vi "Get_Length_of_Tracks-2.vi"(0 "[IN] Grouped Tracks":dbl[][](array[numeric])) -> (1 "[OUT] Tracks Length\nin the Group":u16[](array[numeric]), 2 "[OUT] Single duration \ntrack exists in this\ngroup of tracks":bool, 3 "[OUT] Indexes of single \nframe tracks in the group":i32[](array[numeric]))   [LabVIEW 2013]
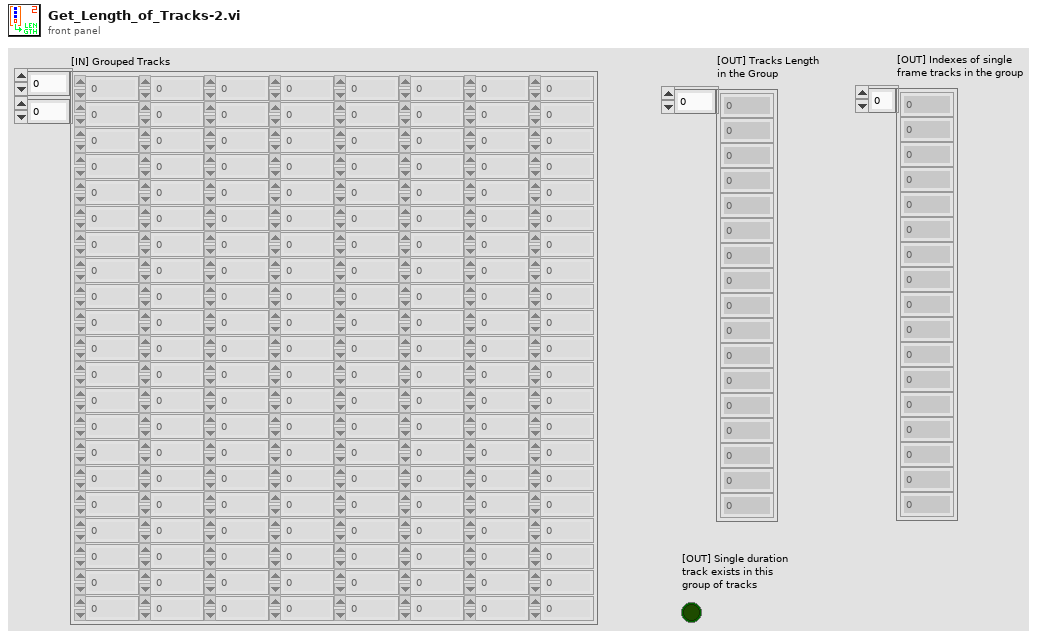
[diagram p1: front panel]
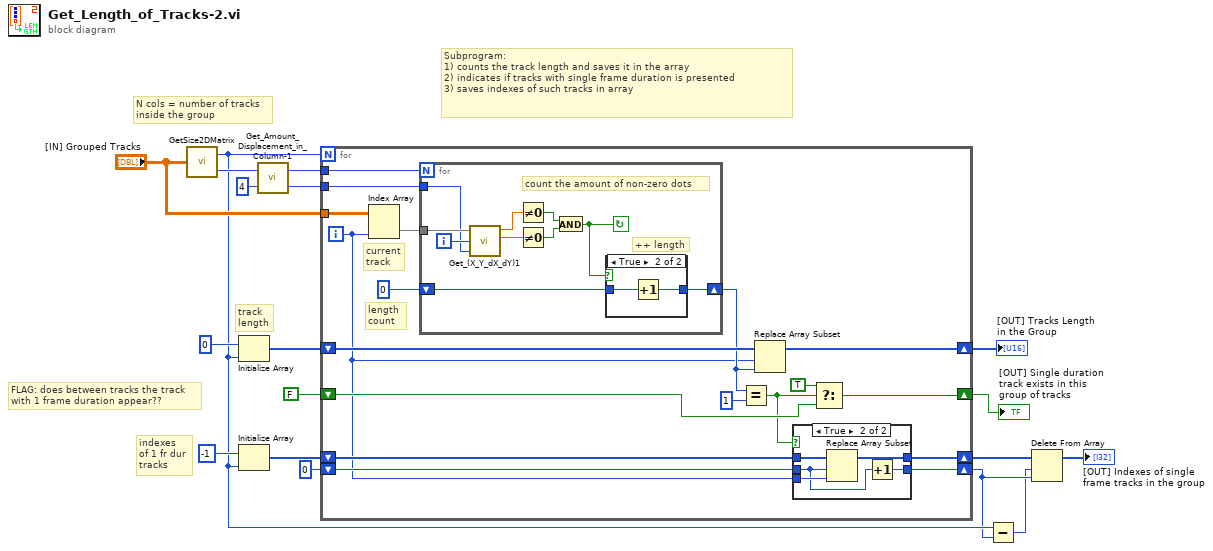
[diagram p0: block diagram]
diagram:
  # "Subprogram: \n1) counts the track length and saves it in the array\n2) indicates if tracks with single frame duration is presented\n3) saves indexes of such tracks in array"
  # "indexes \nof 1 fr dur\ntracks"
  # "FLAG: does between tracks the track \nwith 1 frame duration appear??"
  # "track \nlength"
  # "N cols = number of tracks \ninside the group"
  n1 = call "GetSize2DMatrix.vi"("Array IN (2D)"="[IN] Grouped Tracks") -> ("# Cols"=w4:i32, "# Rows"=w16:i32)
  n2 = Initialize Array(u16 0 ("element"), w4) -> (w17:u16[])
  n3 = Initialize Array(-1 ("element"), w4) -> (w8:i32[])
  n4 = call "Get_Amount_Displacement_in_Column-1.vi"("multiplier"=4, "# Rows"=w16) -> ("multiplier out"=w13:i32, "Displ amount"=w14:i32)
  n5 = for {
    N: w4 -> [_]
    tunnel: "[IN] Grouped Tracks" -> [w36]
    shift-right: [w30] -> w11
    shift-left: w17 -> [w31]
    tunnel: w14 -> [w35]
    tunnel: w13 -> [w34]
    shift-right: [w25] -> w10
    shift-left: FALSE -> [w27]
    shift-right: [w19] -> w5
    shift-left: w8 -> [w23]
    shift-right: [w20] -> w3
    shift-left: 0 -> [w22]
    i -> [w21]
    # "length \ncount"
    # "current\ntrack"
    n6 = Index Array(array=w36, index (col)=w21) -> (element=w33:dbl[])  [unwired: 1 in]
    n7 = for {
      N: w35 -> [_]
      tunnel: w34 -> [w51]
      tunnel: w33 -> [w53]
      shift-right: [w44] -> w29
      shift-left: u16 0 ("element") -> [w45]
      i -> [w52]
      stop <- w46 continue-if-true
      # "++ length"
      # "count the amount of non-zero dots"
      n8 = call "Get_(X_Y_dX_dY)1.vi"("(X,Y,dX,dY)"=w53, "index"=w52, "multiplier"=w51) -> ("X"=w50:dbl, "Y"=w49:dbl)  [unwired: 2 out]
      n9 = Not Equal To 0?(x=w50) -> (x != 0?=w48:bool)
      n10 = Not Equal To 0?(x=w49) -> (x != 0?=w47:bool)
      n11 = And(x=w48, y=w47) -> (x .and. y?=w46:bool)
      n12 = case shown="True" w46 {
        tunnel: w45 -> [w54 w56]
        tunnel: [w54 w55] -> w44
        frame False {
        }
        frame True {
          n13 = Increment(x=w56) -> (x+1=w55:u16)
        }
      }
    }
    n14 = Equal?(x=w29, y=u16 1) -> (x = y?=w24:bool)
    n15 = Replace Array Subset(array=w31, new element=w29, index=w21) -> (w30:u16[])
    n16 = case shown="True" w24 {
      tunnel: w23 -> [w38 w43]
      tunnel: w22 -> [w37 w41]
      tunnel: w21 -> [_ w42]
      tunnel: [w37 w40] -> w20
      tunnel: [w38 w39] -> w19
      frame False {
      }
      frame True {
        n17 = Replace Array Subset(array=w43, new element=w42, index=w41) -> (w39:i32[])
        n18 = Increment(x=w41) -> (x+1=w40:i32)
      }
    }
    n19 = Select(t=TRUE, s=w24, f=w27) -> (s? t:f=w25:bool)
  }
  "[OUT] Tracks Length\nin the Group" <- w11
  "[OUT] Single duration \ntrack exists in this\ngroup of tracks" <- w10
  n20 = Subtract(x=w4, y=w3) -> (x-y=w2:i32)
  n21 = Delete From Array(array=w5, length=w2, index=w3) -> (array with subset deleted=→"[OUT] Indexes of single \nframe tracks in the group":i32[])  [unwired: 1 out]
